vi "Charact One Point.vi"(0 "Scalar SA Path in":refnum<class "SA Path.lvclass">, 5 "Cal point in":T1, 11 "error in (no error)":errorcluster) -> (4 "Scalar SA Path out":refnum<class "SA Path.lvclass">, 15 "error out":errorcluster)   [LabVIEW 2023, in "RFFixtureCharact.Public.lvlib" / "SA Path.lvclass"]
uses:
  SA Path.lvclass
  Scalar Path/Type Definitions/Cal Point.ctl
  SA Abstract Path/SA Abstract Path.lvclass
  Scalar Path/Scalar Path.lvclass
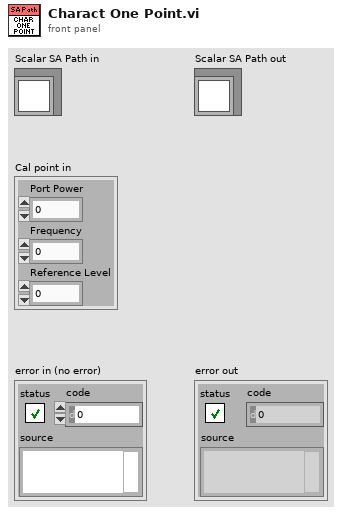
[diagram p1: front panel]
types:
  T1 = typedef "RFFixtureCharact.Public.lvlib/Scalar Path.lvclass/Cal Point.ctl" = cluster{"Port Power":dbl, "Frequency":dbl, "Reference Level":dbl}
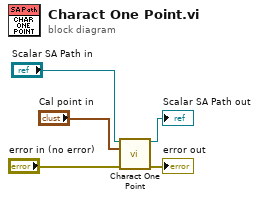
[diagram p0: block diagram]
diagram:
  n1 = call-parent "Charact One Point.vi"("Scalar SA Path in"="Scalar SA Path in", "Cal point in"="Cal point in", "error in (no error)"="error in (no error)") -> ("Scalar SA Path out"=→"Scalar SA Path out":refnum<class "SA Path.lvclass">, "error out"=→"error out":errorcluster)  [unwired: 11 in]
